vi "SettingVariable.vi"() -> ()   [LabVIEW 2020]
panel:
  in  "电压脉冲卡":tag
  in  "波特率":u32
  in  "串口电流服务 2":string
  in  "串口电流服务 1":string
  in  "电压脉冲开关":bool
  in  "电流表串口 2":string
  in  "电流表串口 1":string
  in  "source":dbl
  in  "lifetime":dbl
  in  "lambda":dbl[](array[numeric])
  in  "beta":dbl[](array[numeric])
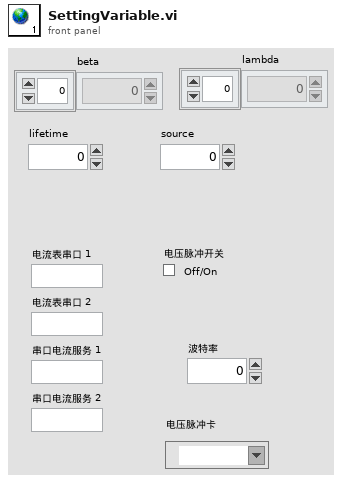
[diagram p1: front panel]
diagram:
